vi "Menu Button - Update Colors.vi"(5 "Header In":refnum<vi>, 7 "RadioButtonsControl in":refnum<vi>, 11 "Display State In in":T1={"Header"="", "Label[]"=[], "DisableButtonsLUT"=variant(string[] []), "Menu Config"=variant}) -> (3 "Display State In out":T1={"Header"="", "Label[]"=[], "DisableButtonsLUT"=variant(string[] []), "Menu Config"=variant})   [LabVIEW 2019, in "Menu Button.xctl"]
doc: "JSMA Module Template - Top Level UI 0.2.0.4\nRob Humfeld - Jet Engineering\nCopyright (c) 2019, Jet Engineering"
uses:
  Menu Button.xctl
  State 1.ctl
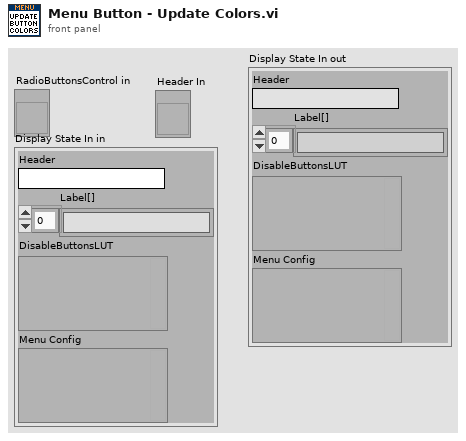
[diagram p1: front panel]
types:
  T1 = typedef "Menu Button.xctl/State 1.ctl" = cluster{"Header":string, "Label[]":string[], "DisableButtonsLUT":variant, "Menu Config":variant}
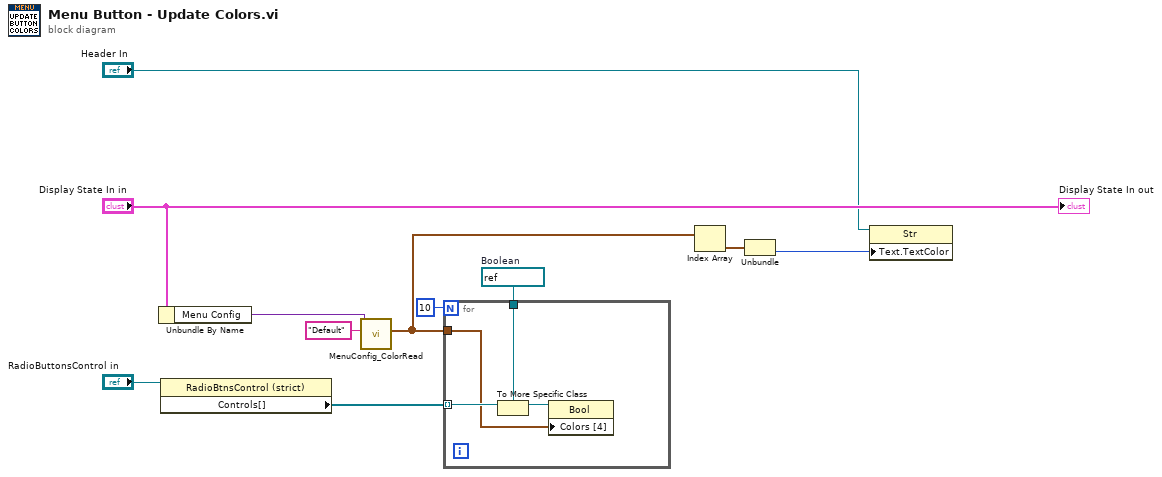
[diagram p0: block diagram]
diagram:
  w11 = refnum<vi> refnum  # Boolean
  n1 = Unbundle By Name("Display State In in") -> ("Menu Config"=w3:variant)
  n2 = property on="Property Node" class="RadioBtnsControl (strict)"(reference="RadioButtonsControl in") -> ("Controls[]"=w10:refnum<vi>[])  [unwired: 1 in, 2 out]
  n3 = call "MenuConfig_ColorRead.vi"("Color.Name (\"Default\")"="Default" ("Color.Name (\"Default\")"), "MenuConfig"=w3) -> ("Colors[4]"=w1:cluster{u32, u32}[])  [unwired: 7 in, 2 out]
  n4 = for {
    N: 10 -> [_]
    tunnel: w10 -> [w15] mode=indexing
    tunnel: w11 -> [w13]
    tunnel: w1 -> [w12]
    n5 = To More Specific Class(target class=w13, reference=w15) -> (specific class reference=w14:refnum<vi>)  [unwired: 1 in, 1 out]
    n6 = property class="Bool"(reference=w14, "Colors [4]"=w12) -> ()  [unwired: 1 in, 2 out]
  }
  n7 = Index Array(array=w1) -> (element=w6:cluster{u32, u32})  [unwired: 1 in]
  n8 = Unbundle(w6) -> (w4:u32)  [unwired: 1 out]
  n9 = property class="Str"(reference="Header In", "Text.TextColor"=w4) -> ()  [unwired: 1 in, 2 out]
  "Display State In out" <- "Display State In in"
